vi "Increment Score.vi"(8 "error in (no error)":errorcluster, 10 "Points Awarded":i32, 11 "Contestant in":refnum<class "Contestant.lvclass">) -> (0 "error out":errorcluster, 3 "Contestant out":refnum<class "Contestant.lvclass">)   [LabVIEW 2021, in "Contestant.lvlib" / "Contestant.lvclass"]
uses:
  Contestant.lvclass
  Contestant.lvclass/Contestant.ctl
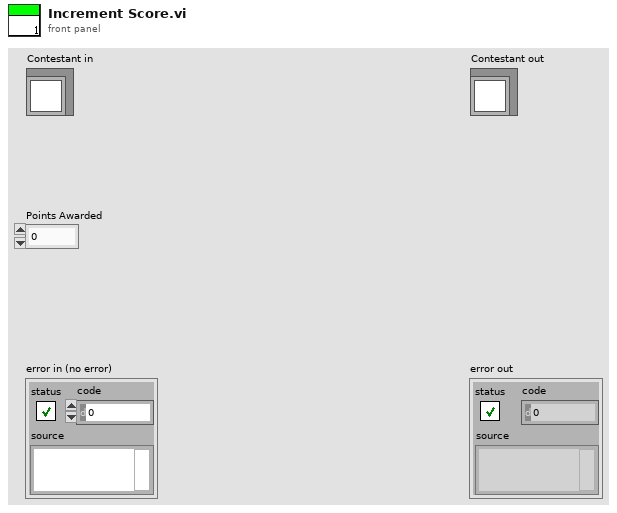
[diagram p1: front panel]
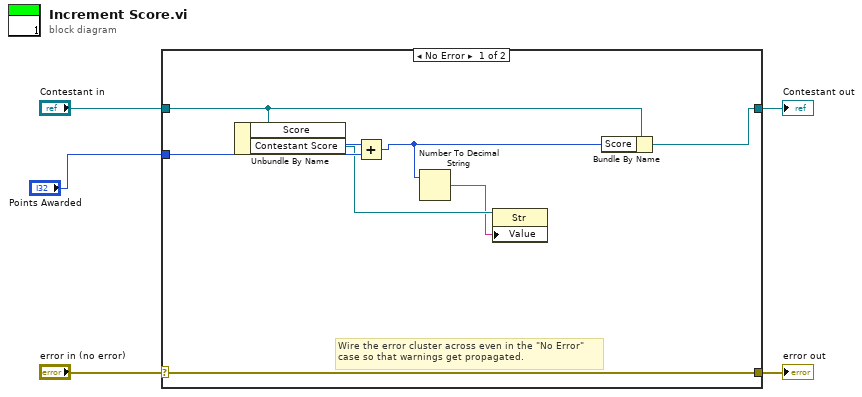
[diagram p0: block diagram]
diagram:
  n1 = case shown="No Error" "error in (no error)" {
    selector: "error in (no error)" -> [w13 w15]
    tunnel: [w13 w15] -> w4
    tunnel: [w9 w14] -> w2
    tunnel: "Contestant in" -> [w10 w14]
    tunnel: "Points Awarded" -> [w11 _]
    frame No Error {
      # "Wire the error cluster across even in the \"No Error\"\ncase so that warnings get propagated."
      n2 = Unbundle By Name(w10) -> ("Score"=w12:i32, "Contestant Score"=w8:refnum<vi>)
      n3 = Add(x=w12, y=w11) -> (x+y=w7:i32)
      n4 = Number To Decimal String(number=w7) -> (decimal integer string=w6:string)  [unwired: 1 in]
      n5 = property class="Str"(reference=w8, "Value"=w6) -> ()  [unwired: 1 in, 2 out]
      n6 = Bundle By Name(cluster=w10, "Score"=w7) -> (w9:refnum<class "Contestant.lvclass">)
    }
    frame Error {
    }
  }
  "error out" <- w4
  "Contestant out" <- w2
